vi "读取CH2.vi"(2 "终止点数":i32, 3 "起始点数":i32, 4 "VISA resource name":refnum<visa-resource-name>) -> (1 "Waveform":dbl[](graph))   [LabVIEW 2018]
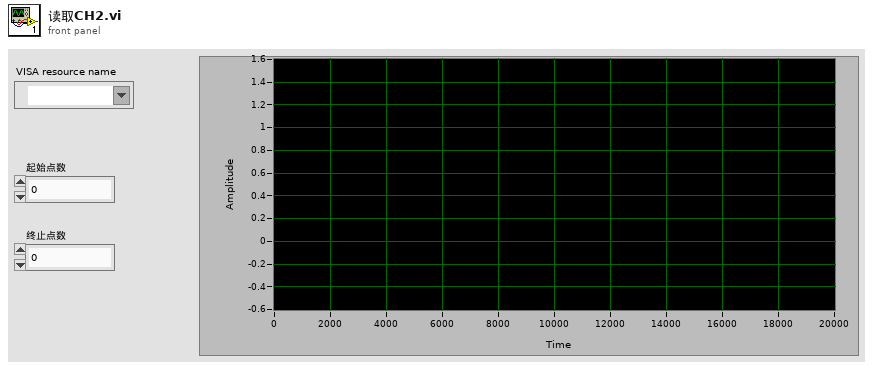
[diagram p1: front panel]
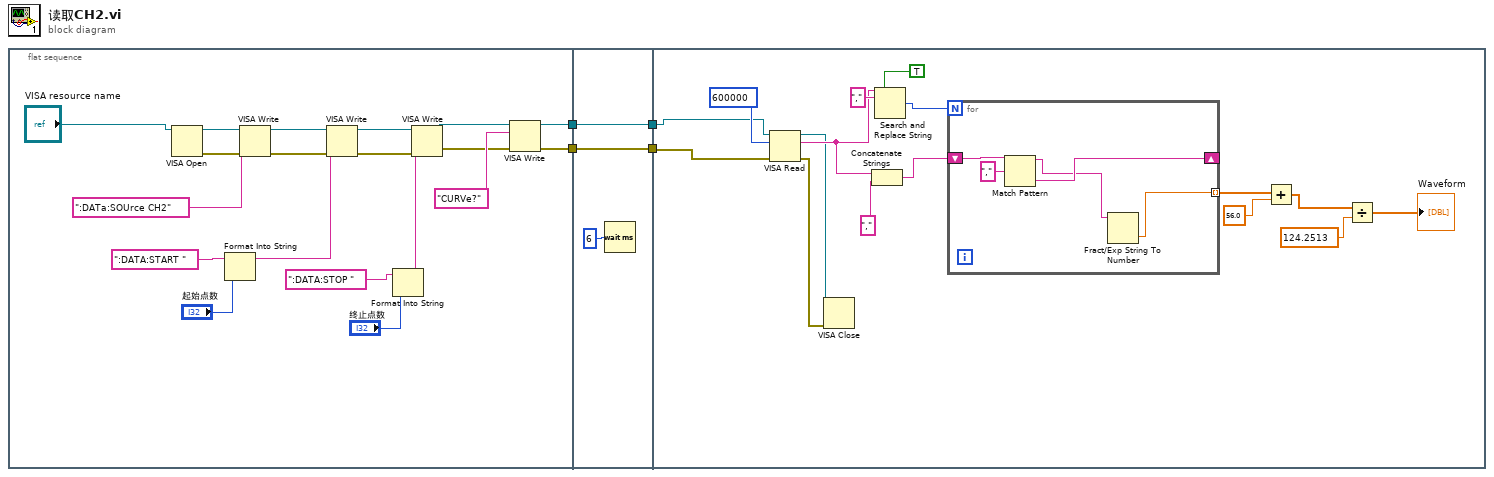
[diagram p0: block diagram]
diagram:
  n1 = flat-sequence {
    tunnel: [w20] -> w4
    tunnel: [w19] -> w3
    tunnel: w4 -> [w26]
    tunnel: w3 -> [w25]
    tunnel: [w26] -> w2
    tunnel: [w25] -> w1
    tunnel: w2 -> [w33]
    tunnel: w1 -> [w32]
    frame #0 {
      n2 = VISA Open(VISA resource name="VISA resource name") -> (VISA resource name=w13:refnum<visa-resource-name>, error out=w12:errorcluster)  [unwired: 4 in]
      n3 = Format Into String(initial string=":DATA:START " ("写入缓冲区"), "起始点数") -> (resulting string=w8:string)  [unwired: 2 in, 1 out]
      n4 = VISA Write(VISA resource name=w13, write buffer=":DATa:SOUrce CH2" ("写入缓冲区"), error in (no error)=w12) -> (VISA resource name out=w18:refnum<visa-resource-name>, error out=w17:errorcluster)  [unwired: 1 out]
      n5 = VISA Write(VISA resource name=w18, write buffer=w8, error in (no error)=w17) -> (VISA resource name out=w16:refnum<visa-resource-name>, error out=w15:errorcluster)  [unwired: 1 out]
      n6 = Format Into String(initial string=":DATA:STOP " ("写入缓冲区"), "终止点数") -> (resulting string=w5:string)  [unwired: 2 in, 1 out]
      n7 = VISA Write(VISA resource name=w16, write buffer=w5, error in (no error)=w15) -> (VISA resource name out=w22:refnum<visa-resource-name>, error out=w21:errorcluster)  [unwired: 1 out]
      n8 = VISA Write(VISA resource name=w22, write buffer="CURVe?", error in (no error)=w21) -> (VISA resource name out=w20:refnum<visa-resource-name>, error out=w19:errorcluster)  [unwired: 1 out]
    }
    frame #1 {
      n9 = Wait (ms)(milliseconds to wait=u32 6 ("等待时间（毫秒）")) -> ()  [unwired: 1 out]
    }
    frame #2 {
      n10 = VISA Read(VISA resource name=w33, byte count=u32 600000, error in (no error)=w32) -> (VISA resource name out=w35:refnum<visa-resource-name>, read buffer=w36:string, error out=w34:errorcluster)  [unwired: 1 out]
      n11 = VISA Close(VISA resource name=w35, error in (no error)=w34) -> ()  [unwired: 1 out]
      n12 = Concatenate Strings(w36, "," ("字符串")) -> (w39:string)
      n13 = Search and Replace String(replace all?=TRUE ("替换全部？(F)"), input string=w36, search string="," ("搜索字符串")) -> (number of replacements=w41:i32)  [unwired: 5 in, 3 out]
      n14 = for {
        N: w41 -> [_]
        shift-right: [w45] -> _
        shift-left: w39 -> [w47]
        tunnel: [w44] -> w31 mode=indexing
        n15 = Match Pattern(string=w47, regular expression="," ("正则表达式")) -> (before substring=w43:string, after substring=w45:string)  [unwired: 1 in, 2 out]
        n16 = Fract/Exp String To Number(string=w43) -> (number=w44:dbl)  [unwired: 3 in, 1 out]
      }
      n17 = Add(x=w31, y=56.0) -> (x+y=w28:dbl[])
      n18 = Divide(x=w28, y=124.2513) -> (x/y=→"Waveform":dbl[])
    }
  }
